vi "DMSO_transfer_sample_to_cell.vi"(6 "COM Port":refnum<visa-resource-name>="COM7", 7 "Pump Parameters":T1={"Speed 1"="100", "Speed 2"="250", "Speed 3"="250", "Speed 4"="250", "UW/Sample"="5", "Sparge"="2", "Std"="4", "Waste"="15", "Air"="14", "Milli-Q"="1", "H2SO4"="6", "NaOH"="3", "Catalyst"="7", "Cell (H+ side)"="8", "Cell (sample side)"="9", "NaCl"="9"}, 8 "step to ml":dbl=1920.0, 10 "Sample Vol. (mL)":dbl, 11 "Extra Milli-Q (ml)":dbl=4.0) -> ()   [LabVIEW 2021]
panel:
  out "Full Command":string="V100O1P7680O9D7680"
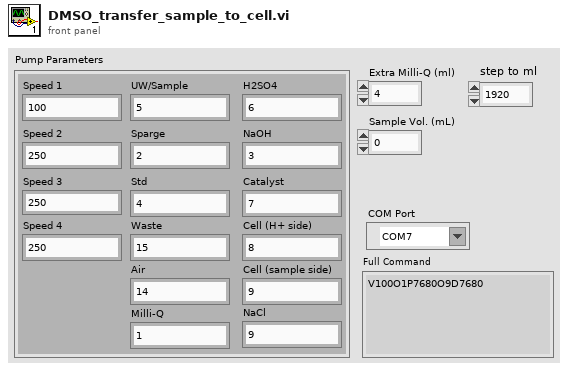
[diagram p1: front panel]
types:
  T1 = cluster{"Speed 1":string, "Speed 2":string, "Speed 3":string, "Speed 4":string, "UW/Sample":string, "Sparge":string, "Std":string, "Waste":string, "Air":string, "Milli-Q":string, "H2SO4":string, "NaOH":string, "Catalyst":string, "Cell (H+ side)":string, "Cell (sample side)":string, "NaCl":string}
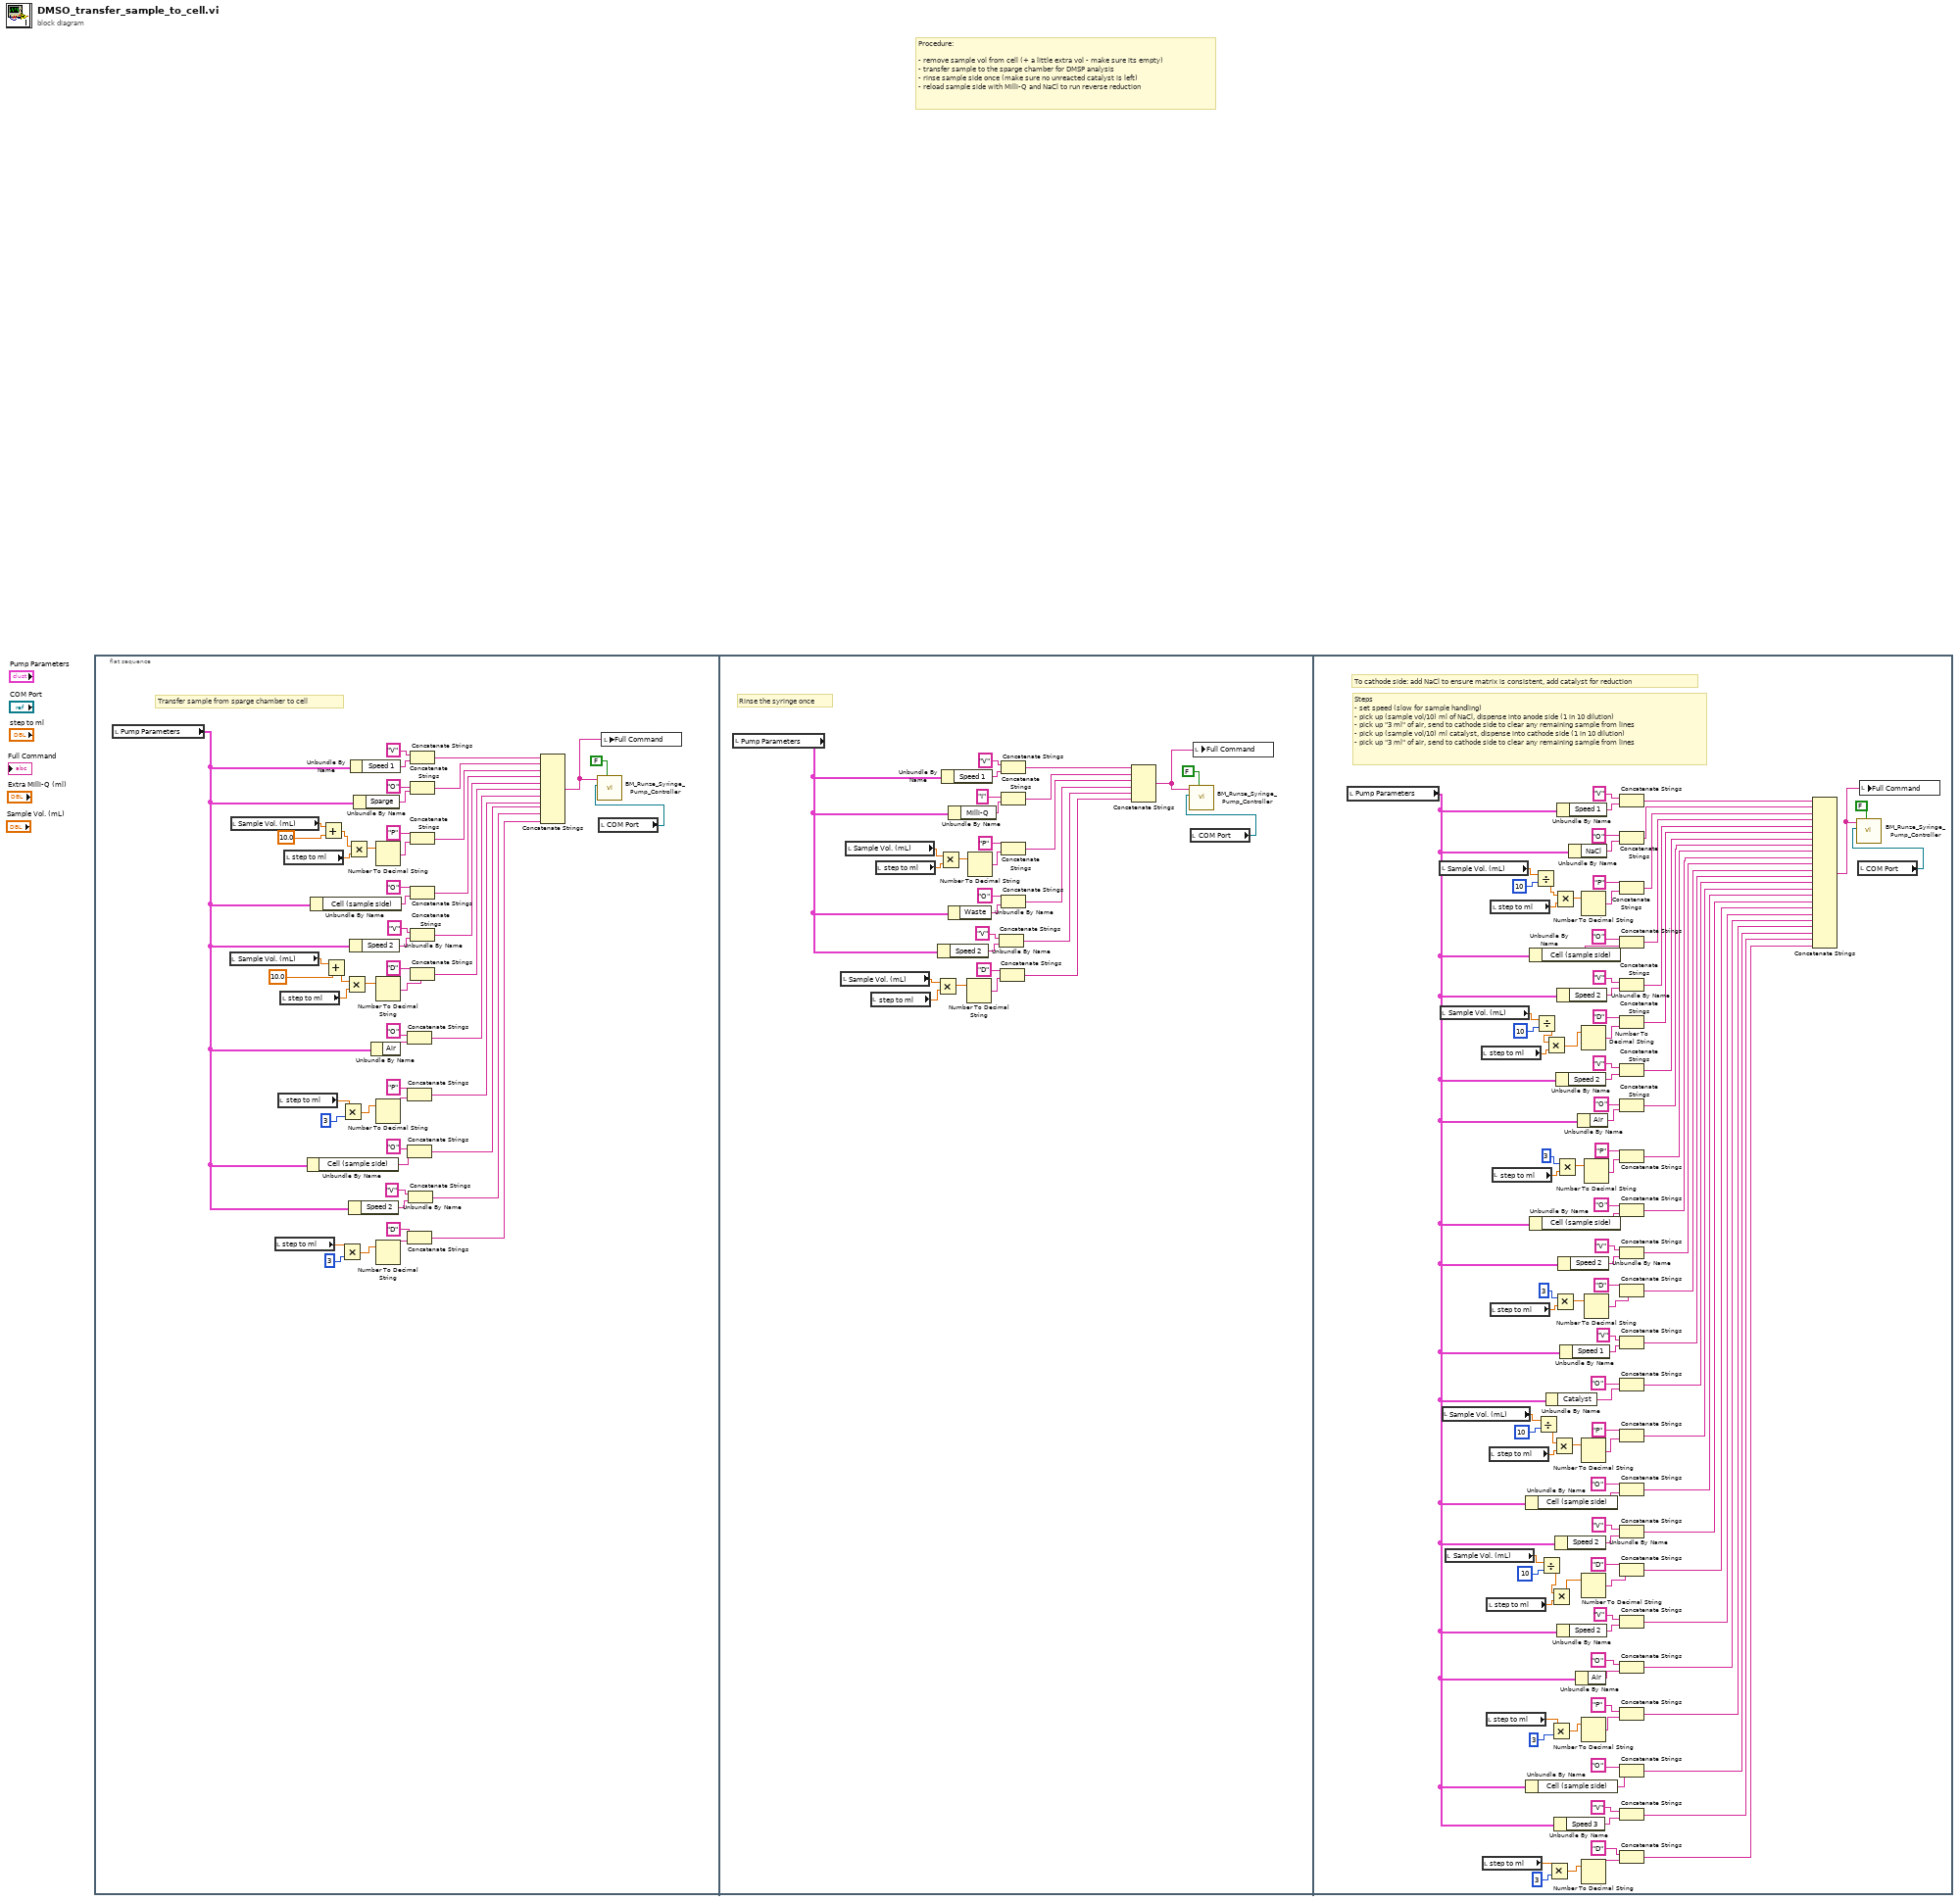
[diagram p0: block diagram]
diagram:
  # "Procedure:\n\n- remove sample vol from cell (+ a little extra vol - make sure its empty)\n- transfer sample to the sparge chamber for DMSP analysis\n- rinse sample side once (make sure no unreacted catalyst is left)\n- reload sample side with Milli-Q and NaCl to run reverse reduction"
  n1 = flat-sequence {
    frame #0 {
      # "Transfer sample from sparge chamber to cell"
      n2 = local read "Pump Parameters"() -> (w6:T1)
      n3 = local read "Sample Vol. (mL)"() -> (w25:dbl)
      n4 = local read "Sample Vol. (mL)"() -> (w28:dbl)
      n5 = local read "step to ml"() -> (w16:dbl)
      n6 = local read "step to ml"() -> (w11:dbl)
      n7 = local read "step to ml"() -> (w44:dbl)
      n8 = local read "step to ml"() -> (w49:dbl)
      n9 = Unbundle By Name(w6) -> ("Cell (sample side)"=w13:string)
      n10 = Unbundle By Name(w6) -> ("Cell (sample side)"=w29:string)
      n11 = Add(x=w28, y=10.0) -> (x+y=w26:dbl)
      n12 = Add(x=w25, y=10.0) -> (x+y=w23:dbl)
      n13 = Multiply(x=w16, y=3) -> (x*y=w15:dbl)
      n14 = Multiply(x=w11, y=3) -> (x*y=w7:dbl)
      n15 = Multiply(x=w23, y=w44) -> (x*y=w45:dbl)
      n16 = Multiply(x=w26, y=w49) -> (x*y=w50:dbl)
      n17 = Unbundle By Name(w6) -> ("Speed 2"=w21:string)
      n18 = Unbundle By Name(w6) -> ("Speed 2"=w34:string)
      n19 = Unbundle By Name(w6) -> ("Speed 1"=w51:string)
      n20 = Unbundle By Name(w6) -> ("Sparge"=w30:string)
      n21 = Unbundle By Name(w6) -> ("Air"=w12:string)
      n22 = Number To Decimal String(number=w50) -> (decimal integer string=w47:string)  [unwired: 1 out]
      n23 = Number To Decimal String(number=w45) -> (decimal integer string=w42:string)  [unwired: 1 out]
      n24 = Number To Decimal String(number=w7) -> (decimal integer string=w18:string)  [unwired: 1 out]
      n25 = Number To Decimal String(number=w15) -> (decimal integer string=w20:string)  [unwired: 1 out]
      n26 = Concatenate Strings("O", w12) -> (w5:string)
      n27 = Concatenate Strings("P", w18) -> (w4:string)
      n28 = Concatenate Strings("O", w13) -> (w3:string)
      n29 = Concatenate Strings("D", w20) -> (w1:string)
      n30 = Concatenate Strings("V", w21) -> (w2:string)
      n31 = Concatenate Strings("V", w51) -> (w41:string)
      n32 = Concatenate Strings("O", w30) -> (w40:string)
      n33 = Concatenate Strings("P", w47) -> (w39:string)
      n34 = Concatenate Strings("O", w29) -> (w38:string)
      n35 = Concatenate Strings("D", w42) -> (w32:string)
      n36 = Concatenate Strings("V", w34) -> (w33:string)
      n37 = Concatenate Strings(w41, w40, w39, w38, w33, w32, w5, w4, w3, w2, w1) -> (w37:string)
      n38 = local read "COM Port"() -> (w36:refnum<visa-resource-name>)
      n39 = call "BM_Runze_Syringe_Pump_Controller.vi"("Initialize Plunger?"=FALSE ("Initialize?"), "COM Port (Runze)"=w36, "Enter Command"=w37) -> ()  [unwired: 6 in, 3 out]
      n40 = local write "Full Command"(w37) -> ()
    }
    frame #1 {
      # "Rinse the syringe once"
      n41 = local read "Pump Parameters"() -> (w54:T1)
      n42 = local read "Sample Vol. (mL)"() -> (w64:dbl)
      n43 = local read "Sample Vol. (mL)"() -> (w68:dbl)
      n44 = local read "step to ml"() -> (w62:dbl)
      n45 = local read "step to ml"() -> (w73:dbl)
      n46 = Multiply(x=w64, y=w62) -> (x*y=w63:dbl)
      n47 = Unbundle By Name(w54) -> ("Speed 2"=w58:string)
      n48 = Multiply(x=w68, y=w73) -> (x*y=w72:dbl)
      n49 = Unbundle By Name(w54) -> ("Speed 1"=w71:string)
      n50 = Unbundle By Name(w54) -> ("Waste"=w65:string)
      n51 = Unbundle By Name(w54) -> ("Milli-Q"=w67:string)
      n52 = Number To Decimal String(number=w63) -> (decimal integer string=w60:string)  [unwired: 1 out]
      n53 = Number To Decimal String(number=w72) -> (decimal integer string=w75:string)  [unwired: 1 out]
      n54 = Concatenate Strings("V", w58) -> (w56:string)
      n55 = Concatenate Strings("D", w60) -> (w55:string)
      n56 = Concatenate Strings("V", w71) -> (w76:string)
      n57 = Concatenate Strings("I", w67) -> (w77:string)
      n58 = Concatenate Strings("P", w75) -> (w78:string)
      n59 = Concatenate Strings("O", w65) -> (w57:string)
      n60 = Concatenate Strings(w76, w77, w78, w57, w56, w55) -> (w79:string)
      n61 = local read "COM Port"() -> (w80:refnum<visa-resource-name>)
      n62 = call "BM_Runze_Syringe_Pump_Controller.vi"("Initialize Plunger?"=FALSE ("Initialize?"), "COM Port (Runze)"=w80, "Enter Command"=w79) -> ()  [unwired: 6 in, 3 out]
      n63 = local write "Full Command"(w79) -> ()
    }
    frame #2 {
      # "Steps\n- set speed (slow for sample handling)\n- pick up (sample vol/10) ml of NaCl, dispense into anode side (1 in 10 dilution)\n- pick up \"3 ml\" of air, send to cathode side to clear any remaining sample from lines\n- pick up (sample vol/10) ml catalyst, dispense into cathode side (1 in 10 dilution)\n- pick up \"3 ml\" of air, send to cathode side to clear any remaining sample from lines"
      # "To cathode side: add NaCl to ensure matrix is consistent, add catalyst for reduction"
      n64 = local read "Pump Parameters"() -> (w177:T1)
      n65 = local read "Sample Vol. (mL)"() -> (w178:dbl)
      n66 = local read "Sample Vol. (mL)"() -> (w182:dbl)
      n67 = local read "Sample Vol. (mL)"() -> (w184:dbl)
      n68 = local read "Sample Vol. (mL)"() -> (w187:dbl)
      n69 = local read "step to ml"() -> (w125:dbl)
      n70 = local read "step to ml"() -> (w105:dbl)
      n71 = local read "step to ml"() -> (w100:dbl)
      n72 = local read "step to ml"() -> (w92:dbl)
      n73 = local read "step to ml"() -> (w86:dbl)
      n74 = local read "step to ml"() -> (w149:dbl)
      n75 = local read "step to ml"() -> (w119:dbl)
      n76 = local read "step to ml"() -> (w142:dbl)
      n77 = Unbundle By Name(w177) -> ("Cell (sample side)"=w90:string)
      n78 = Unbundle By Name(w177) -> ("Cell (sample side)"=w101:string)
      n79 = Unbundle By Name(w177) -> ("Cell (sample side)"=w123:string)
      n80 = Unbundle By Name(w177) -> ("Cell (sample side)"=w146:string)
      n81 = Divide(x=w178, y=10) -> (x/y=w180:dbl)
      n82 = Divide(x=w182, y=10) -> (x/y=w183:dbl)
      n83 = Divide(x=w184, y=10) -> (x/y=w188:dbl)
      n84 = Divide(x=w187, y=10) -> (x/y=w189:dbl)
      n85 = Multiply(x=w183, y=w125) -> (x*y=w124:dbl)
      n86 = Unbundle By Name(w177) -> ("Catalyst"=w109:string)
      n87 = Multiply(x=w105, y=3) -> (x*y=w104:dbl)
      n88 = Multiply(x=w100, y=3) -> (x*y=w97:dbl)
      n89 = Multiply(x=w189, y=w92) -> (x*y=w91:dbl)
      n90 = Multiply(x=w188, y=w86) -> (x*y=w85:dbl)
      n91 = Multiply(x=3, y=w149) -> (x*y=w148:dbl)
      n92 = Multiply(x=w180, y=w119) -> (x*y=w118:dbl)
      n93 = Unbundle By Name(w177) -> ("Speed 3"=w176:string)
      n94 = Multiply(x=3, y=w142) -> (x*y=w141:dbl)
      n95 = Unbundle By Name(w177) -> ("Speed 2"=w113:string)
      n96 = Unbundle By Name(w177) -> ("Speed 2"=w157:string)
      n97 = Unbundle By Name(w177) -> ("Speed 1"=w84:string)
      n98 = Unbundle By Name(w177) -> ("Speed 2"=w129:string)
      n99 = Unbundle By Name(w177) -> ("Speed 2"=w158:string)
      n100 = Unbundle By Name(w177) -> ("Speed 2"=w153:string)
      n101 = Unbundle By Name(w177) -> ("Speed 1"=w155:string)
      n102 = Unbundle By Name(w177) -> ("NaCl"=w131:string)
      n103 = Unbundle By Name(w177) -> ("Air"=w96:string)
      n104 = Unbundle By Name(w177) -> ("Air"=w156:string)
      n105 = Number To Decimal String(number=w85) -> (decimal integer string=w88:string)  [unwired: 1 out]
      n106 = Number To Decimal String(number=w91) -> (decimal integer string=w94:string)  [unwired: 1 out]
      n107 = Number To Decimal String(number=w97) -> (decimal integer string=w103:string)  [unwired: 1 out]
      n108 = Number To Decimal String(number=w104) -> (decimal integer string=w108:string)  [unwired: 1 out]
      n109 = Number To Decimal String(number=w118) -> (decimal integer string=w121:string)  [unwired: 1 out]
      n110 = Number To Decimal String(number=w124) -> (decimal integer string=w127:string)  [unwired: 1 out]
      n111 = Number To Decimal String(number=w141) -> (decimal integer string=w144:string)  [unwired: 1 out]
      n112 = Number To Decimal String(number=w148) -> (decimal integer string=w151:string)  [unwired: 1 out]
      n113 = Concatenate Strings("V", w84) -> (w132:string)
      n114 = Concatenate Strings("O", w131) -> (w133:string)
      n115 = Concatenate Strings("P", w121) -> (w134:string)
      n116 = Concatenate Strings("O", w123) -> (w135:string)
      n117 = Concatenate Strings("V", w129) -> (w136:string)
      n118 = Concatenate Strings("D", w127) -> (w137:string)
      n119 = Concatenate Strings("V", w157) -> (w138:string)
      n120 = Concatenate Strings("O", w156) -> (w159:string)
      n121 = Concatenate Strings("P", w144) -> (w160:string)
      n122 = Concatenate Strings("O", w146) -> (w161:string)
      n123 = Concatenate Strings("V", w153) -> (w162:string)
      n124 = Concatenate Strings("D", w151) -> (w163:string)
      n125 = Concatenate Strings("V", w155) -> (w164:string)
      n126 = Concatenate Strings("O", w109) -> (w165:string)
      n127 = Concatenate Strings("P", w88) -> (w166:string)
      n128 = Concatenate Strings("O", w90) -> (w167:string)
      n129 = Concatenate Strings("V", w113) -> (w168:string)
      n130 = Concatenate Strings("D", w94) -> (w169:string)
      n131 = Concatenate Strings("V", w158) -> (w170:string)
      n132 = Concatenate Strings("O", w96) -> (w171:string)
      n133 = Concatenate Strings("P", w103) -> (w172:string)
      n134 = Concatenate Strings("O", w101) -> (w173:string)
      n135 = Concatenate Strings("V", w176) -> (w174:string)
      n136 = Concatenate Strings("D", w108) -> (w175:string)
      n137 = Concatenate Strings(w132, w133, w134, w135, w136, w137, w138, w159, w160, w161, w162, w163, w164, w165, w166, w167, w168, w169, w170, w171, w172, w173, w174, w175) -> (w111:string)
      n138 = local read "COM Port"() -> (w110:refnum<visa-resource-name>)
      n139 = call "BM_Runze_Syringe_Pump_Controller.vi"("Initialize Plunger?"=FALSE ("Initialize?"), "COM Port (Runze)"=w110, "Enter Command"=w111) -> ()  [unwired: 6 in, 3 out]
      n140 = local write "Full Command"(w111) -> ()
    }
  }
